vi "CLSUIP_ReplaceLVClassControls.vi"(8 "error in (no error)":errorcluster, 10 "LVClassLibrary":refnum<vi>, 11 "VI Reference":refnum<vi>) -> (0 "error out":errorcluster, 1 "Indicator Ref":refnum<vi>, 2 "Control Ref":refnum<vi>, 3 "VI Reference out":refnum<vi>)   [LabVIEW 2021, in "MemberVICreation.lvlib"]
uses:
  <resource>/Framework/Providers/LVClassLibrary/NewAccessors/MemberVICreation.lvlib
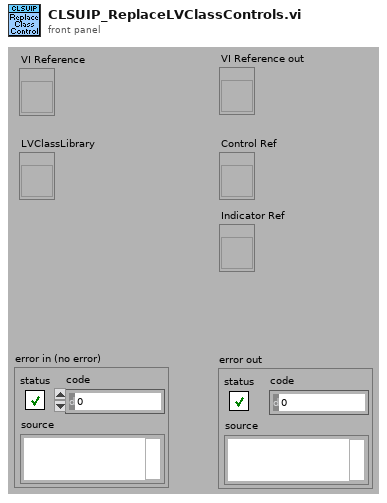
[diagram p1: front panel]
types:
  T1 = typedef "MemberVICreation.lvlib/CLSUIP_ControlInformation.ctl" = cluster{"Indicator":bool, "Position":T2, "Terminal.Position":T2, "Terminal.Icon View?":bool, "TermAssignment":i32, "Connected Terminal":refnum<vi>, "Terminal Owner":refnum<vi>}
  T2 = typedef "LVPositionTypeDef.ctl" = cluster{"Left":i32, "Top":i32}
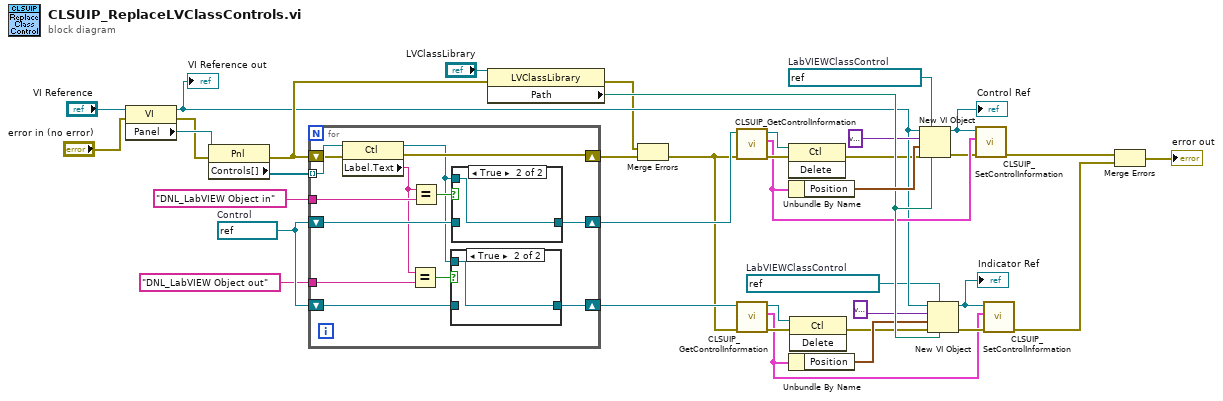
[diagram p0: block diagram]
diagram:
  w2 = refnum<vi> refnum  # LabVIEWClassControl
  w27 = refnum<vi> refnum  # Control
  w20 = refnum<vi> refnum  # LabVIEWClassControl
  n1 = property class="VI"(reference="VI Reference", error in="error in (no error)") -> (reference out=w10:refnum<vi>, error out=w35:errorcluster, "Panel"=w36:refnum<vi>)
  "VI Reference out" <- w10
  n2 = property class="Pnl"(reference=w36, error in=w35) -> (error out=w29:errorcluster, "Controls[]"=w37:refnum<vi>[])  [unwired: 1 out]
  n3 = for {
    tunnel: w37 -> [w51] mode=indexing
    shift-right: [w48] -> w9
    shift-left: w29 -> [w50]
    shift-right: [w47] -> w32
    shift-left: w27 -> [w46]
    shift-right: [w43] -> w25
    shift-left: w27 -> [w40]
    tunnel: "DNL_LabVIEW Object in" ("name") -> [w45]
    tunnel: "DNL_LabVIEW Object out" ("name") -> [w39]
    n4 = property class="Ctl"(reference=w51, error in=w50) -> (reference out=w41:refnum<vi>, error out=w48:errorcluster, "Label.Text"=w42:string)
    n5 = Equal?(x=w42, y=w39) -> (x = y?=w44:bool)
    n6 = Equal?(x=w42, y=w45) -> (x = y?=w49:bool)
    n7 = case shown="True" w44 {
      tunnel: w41 -> [_ w53]
      tunnel: [w52 w53] -> w43
      tunnel: w40 -> [w52 _]
      frame False {
      }
      frame True {
      }
    }
    n8 = case shown="True" w49 {
      tunnel: w41 -> [_ w55]
      tunnel: [w54 w55] -> w47
      tunnel: w46 -> [w54 _]
      frame False {
      }
      frame True {
      }
    }
  }
  n9 = property class="LVClassLibrary"(reference="LVClassLibrary", error in=w29) -> (error out=w8:errorcluster, "Path"=w21:path)  [unwired: 1 out]
  n10 = Merge Errors(w8, w9) -> (w7:errorcluster)
  n11 = call <resource>:"CLSUIP_GetControlInformation.vi"("error in (no error)"=w7, "Ctl Refnum"=w32) -> ("error out"=w30:errorcluster, "Control Information"=w16:T1, "Ctl Refnum out"=w31:refnum<vi>)  [unwired: 7 out]
  n12 = call <resource>:"CLSUIP_GetControlInformation.vi"("error in (no error)"=w7, "Ctl Refnum"=w25) -> ("error out"=w23:errorcluster, "Control Information"=w12:T1, "Ctl Refnum out"=w24:refnum<vi>)  [unwired: 7 out]
  n13 = invoke class="Ctl" method="Delete"(reference=w31, error in=w30) -> (error out=w6:errorcluster)  [unwired: 1 in, 2 out]
  n14 = Unbundle By Name(w16) -> ("Position"=w22:T2)
  n15 = Unbundle By Name(w12) -> ("Position"=w19:T2)
  n16 = invoke class="Ctl" method="Delete"(reference=w24, error in=w23) -> (error out=w5:errorcluster)  [unwired: 1 in, 2 out]
  n17 = New VI Object(vi object class=w20, owner refnum=w10, style=variant, position/next to=w22, 6:w21, 8:w6) -> (object refnum=w17:refnum<vi>, 0:w15:errorcluster)  [unwired: 2 out]
  "Control Ref" <- w17
  n18 = New VI Object(vi object class=w2, owner refnum=w10, style=variant, position/next to=w19, 6:w21, 8:w5) -> (object refnum=w13:refnum<vi>, 0:w14:errorcluster)  [unwired: 2 out]
  "Indicator Ref" <- w13
  n19 = call <resource>:"CLSUIP_SetControlInformation.vi"("error in (no error)"=w15, "Control Information"=w16, "Ctl Refnum"=w17) -> ("error out"=w3:errorcluster)  [unwired: 8 out]
  n20 = call <resource>:"CLSUIP_SetControlInformation.vi"("error in (no error)"=w14, "Control Information"=w12, "Ctl Refnum"=w13) -> ("error out"=w4:errorcluster)  [unwired: 8 out]
  n21 = Merge Errors(w3, w4) -> (→"error out":errorcluster)
